vi "GetColorBoxRect.vi"(8 "error in (no error)":errorcluster caption="错误输入（无错误）", 10 "origin":cluster{"x":i16, "y":i16} caption="原点", 11 "Gradient PieChart 输入":refnum<class "Gradient PieChart.lvclass"> caption="DNL_LabVIEW Object in") -> (0 "error out":errorcluster caption="错误输出", 2 "ColorBoxRect":T1, 3 "Gradient PieChart 输出":refnum<class "Gradient PieChart.lvclass"> caption="DNL_LabVIEW Object out")   [LabVIEW 2012, in "Gradient PieChart.lvclass"]
uses:
  Gradient PieChart.lvclass
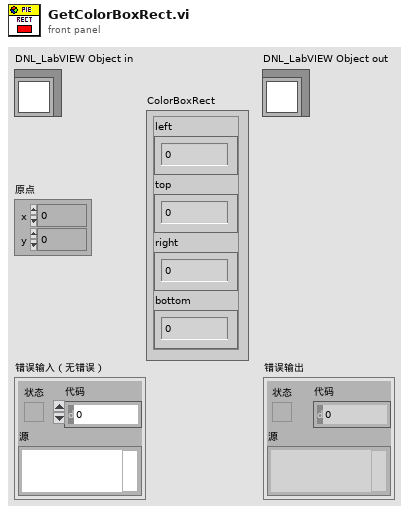
[diagram p1: front panel]
types:
  T1 = cluster{"left":i16, "top":i16, "right":i16, "bottom":i16}
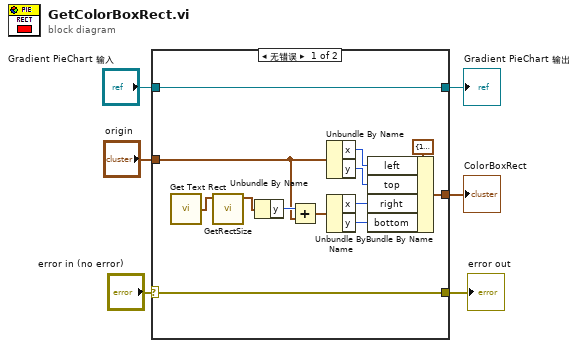
[diagram p0: block diagram]
diagram:
  n1 = case shown="无错误" "error in (no error)" {
    selector: "error in (no error)" -> [w18 w21]
    tunnel: [w18 w21] -> w5
    tunnel: [w19 w20] -> w3
    tunnel: "Gradient PieChart 输入" -> [w19 w20]
    tunnel: "origin" -> [w8 _]
    tunnel: [w7 _] -> w1
    frame No Error {
      n2 = call <vilib>:"Get Text Rect.vi"() -> ("rect"=w9:T1)  [unwired: 9 in]
      n3 = call "GetRectSize.vi"("rect"=w9) -> ("point"=w10:cluster{"x":i16, "y":i16})  [unwired: 7 in, 3 out]
      n4 = Unbundle By Name(w10) -> ("y"=w11:i16)
      n5 = Add(x=w11, y=w8) -> (x+y=w15:cluster{"x":i16, "y":i16})
      n6 = Unbundle By Name(w8) -> ("x"=w13:i16, "y"=w14:i16)
      n7 = Unbundle By Name(w15) -> ("x"=w16:i16, "y"=w17:i16)
      n8 = Bundle By Name(cluster=T1 {"left"=100, "top"=100, "right"=171, "bottom"=117} ("text rect"), "left"=w13, "top"=w14, "right"=w16, "bottom"=w17) -> (w7:T1)
    }
    frame Error {
    }
  }
  "error out" <- w5
  "Gradient PieChart 输出" <- w3
  "ColorBoxRect" <- w1
